vi "UNITEST MAIN v2.0.vi"() -> ()   [LabVIEW 2025] (continued)
      n520 = Bundle By Name(cluster=w613, "New PID LOGIC.Fine Tune Zone"=w611, "New PID LOGIC.PID SDelay"=w610, "New PID LOGIC.Max_pos_limit"=w609, "New PID LOGIC.Min_pos_limit"=w608, "New PID LOGIC.i_limit"=w607, "New PID LOGIC.pct_scale"=w598, "New PID LOGIC.Deadband"=w606, "New PID LOGIC.Kd"=w605, "New PID LOGIC.Ki"=w604, "New PID LOGIC.Kp"=w603, "New PID LOGIC.Current Position"=w602, "New PID LOGIC.Set Load"=w601, "New PID LOGIC.Current Load"=w600, "New PID LOGIC.Pulse delta"=w599, "New PID LOGIC.Init Step"=w597, "New PID LOGIC.Max Step Linit"=w596, "New PID LOGIC.min_deadband_floor"=w595, "New PID LOGIC.dynamic_spindle_noise_scalar"=w594, "New PID LOGIC.min_finetune_floor"=w593, "New PID LOGIC.filter_alpha"=w592, "New PID LOGIC.PID"=w591) -> (w612:T22)
    }
    frame #14 {
      n521 = control-ref of="Manual Write SWAY"() -> (w652:refnum<vi>)
      n522 = control-ref of="Read SWAY Temp"() -> (w633:refnum<vi>)
      n523 = control-ref of="error out Write  SWAY"() -> (w654:refnum<vi>)
      n524 = control-ref of="error out Read SWAY"() -> (w653:refnum<vi>)
      n525 = control-ref of="faultCode Rotary"() -> (w616:refnum<vi>)
      n526 = control-ref of="UPLINK SWAY"() -> (w615:refnum<vi>)
      n527 = control-ref of="DOWNLINK SWAY"() -> (w614:refnum<vi>)
      n528 = control-ref of="fwMajor"() -> (w671:refnum<vi>)
      n529 = control-ref of="Homed"() -> (w670:refnum<vi>)
      n530 = control-ref of="Rotary POSE"() -> (w669:refnum<vi>)
      n531 = control-ref of="State"() -> (w668:refnum<vi>)
      n532 = control-ref of="SWAY POSE"() -> (w667:refnum<vi>)
      n533 = control-ref of="Ack ID"() -> (w666:refnum<vi>)
      n534 = control-ref of="faultCode"() -> (w665:refnum<vi>)
      n535 = control-ref of="Node Id"() -> (w664:refnum<vi>)
      n536 = control-ref of="fwMinor"() -> (w663:refnum<vi>)
      n537 = control-ref of="Spare 6"() -> (w662:refnum<vi>)
      n538 = control-ref of="Spare 5"() -> (w661:refnum<vi>)
      n539 = control-ref of="Spare 4"() -> (w660:refnum<vi>)
      n540 = control-ref of="Spare 3"() -> (w659:refnum<vi>)
      n541 = control-ref of="Spare 2"() -> (w658:refnum<vi>)
      n542 = control-ref of="Spare 1"() -> (w657:refnum<vi>)
      n543 = control-ref of="Spare 7"() -> (w656:refnum<vi>)
      n544 = control-ref of="SPARE  5"() -> (w655:refnum<vi>)
      n545 = control-ref of="SPARE  4"() -> (w650:refnum<vi>)
      n546 = control-ref of="SPARE  3"() -> (w649:refnum<vi>)
      n547 = control-ref of="SPARE 2"() -> (w648:refnum<vi>)
      n548 = control-ref of="SPARE1"() -> (w647:refnum<vi>)
      n549 = control-ref of="Spare 15"() -> (w646:refnum<vi>)
      n550 = control-ref of="Spare 14"() -> (w645:refnum<vi>)
      n551 = control-ref of="Spare 13"() -> (w644:refnum<vi>)
      n552 = control-ref of="Spare 12"() -> (w643:refnum<vi>)
      n553 = control-ref of="Spare 11"() -> (w642:refnum<vi>)
      n554 = control-ref of="Spare 9"() -> (w641:refnum<vi>)
      n555 = control-ref of="Spare 8"() -> (w640:refnum<vi>)
      n556 = control-ref of="SPEED"() -> (w639:refnum<vi>)
      n557 = control-ref of="Distance"() -> (w638:refnum<vi>)
      n558 = control-ref of="Mode Command"() -> (w637:refnum<vi>)
      n559 = control-ref of="Sequence ID"() -> (w636:refnum<vi>)
      n560 = control-ref of="Spare 10"() -> (w634:refnum<vi>)
      n561 = control-ref of="faultCode Sway"() -> (w632:refnum<vi>)
      n562 = control-ref of="Missed Packets"() -> (w631:refnum<vi>)
      n563 = control-ref of="System UPTIME"() -> (w630:refnum<vi>)
      n564 = control-ref of="SPARE 6"() -> (w629:refnum<vi>)
      n565 = control-ref of="SPARE 7"() -> (w628:refnum<vi>)
      n566 = control-ref of="SPARE 9"() -> (w627:refnum<vi>)
      n567 = control-ref of="SPARE 11"() -> (w626:refnum<vi>)
      n568 = control-ref of="SPARE 10"() -> (w625:refnum<vi>)
      n569 = control-ref of="SPARE 8"() -> (w624:refnum<vi>)
      n570 = control-ref of="SPARE 13"() -> (w623:refnum<vi>)
      n571 = control-ref of="SPARE 12"() -> (w622:refnum<vi>)
      n572 = control-ref of="SPARE 17"() -> (w621:refnum<vi>)
      n573 = control-ref of="SPARE 16"() -> (w620:refnum<vi>)
      n574 = control-ref of="SPARE 15"() -> (w619:refnum<vi>)
      n575 = control-ref of="SPARE 14"() -> (w618:refnum<vi>)
      n576 = control-ref of="Reserved"() -> (w617:refnum<vi>)
      n577 = control-ref of="SWAY WRITE"() -> (w651:refnum<vi>)
      n578 = control-ref of="SWAY READ"() -> (w635:refnum<vi>)
      n579 = Bundle By Name(cluster=w673, "SWAY.fwMajor"=w671, "SWAY.Homed"=w670, "SWAY.Rotary POSE"=w669, "SWAY.State"=w668, "SWAY.SWAY POSE"=w667, "SWAY.Ack ID"=w666, "SWAY.faultCode"=w665, "SWAY.Node Id"=w664, "SWAY.fwMinor"=w663, "SWAY.Spare 6"=w662, "SWAY.Spare 5"=w661, "SWAY.Spare 4"=w660, "SWAY.Spare 3"=w659, "SWAY.Spare 2"=w658, "SWAY.Spare 1"=w657, "SWAY.Spare 7"=w656, "SWAY.SPARE  5"=w655, "SWAY.error out Write  SWAY"=w654, "SWAY.error out Read SWAY"=w653, "SWAY.Manual Write SWAY"=w652, "SWAY.SWAY WRITE"=w651, "SWAY.SPARE  4"=w650, "SWAY.SPARE  3"=w649, "SWAY.SPARE 2"=w648, "SWAY.SPARE 1"=w647, "SWAY.Spare 15"=w646, "SWAY.Spare 14"=w645, "SWAY.Spare 13"=w644, "SWAY.Spare 12"=w643, "SWAY.Spare 11"=w642, "SWAY.Spare 9"=w641, "SWAY.Spare 8"=w640, "SWAY.SPEED"=w639, "SWAY.Distance"=w638, "SWAY.Mode Command"=w637, "SWAY.Sequence ID"=w636, "SWAY.SWAY READ"=w635, "SWAY.Spare 10"=w634, "SWAY.Read SWAY Temp"=w633, "SWAY.faultCode Sway"=w632, "SWAY.Missed Packets"=w631, "SWAY.System UPTIME sway"=w630, "SWAY.SPARE 6"=w629, "SWAY.SPARE 7"=w628, "SWAY.SPARE 9"=w627, "SWAY.SPARE 11"=w626, "SWAY.SPARE 10"=w625, "SWAY.SPARE 8"=w624, "SWAY.SPARE 13"=w623, "SWAY.SPARE 12"=w622, "SWAY.SPARE 17"=w621, "SWAY.SPARE 16"=w620, "SWAY.SPARE 15"=w619, "SWAY.SPARE 14"=w618, "SWAY.Reserved"=w617, "SWAY.faultCode Rotary"=w616, "SWAY.UPLINK SWAY"=w615, "SWAY.DOWNLINK SWAY"=w614) -> (w672:T22)
    }
    frame #15 {
      n580 = control-ref of="Analysis Home new"() -> (w704:refnum<vi>)
      n581 = control-ref of="Refresh 2"() -> (w703:refnum<vi>)
      n582 = control-ref of="OPEN 4"() -> (w689:refnum<vi>)
      n583 = control-ref of="OPEN 3"() -> (w687:refnum<vi>)
      n584 = control-ref of="XY Graph"() -> (w682:refnum<vi>)
      n585 = control-ref of="OPEN 2"() -> (w679:refnum<vi>)
      n586 = control-ref of="OPEN 1"() -> (w678:refnum<vi>)
      n587 = control-ref of="Export"() -> (w675:refnum<vi>)
      n588 = control-ref of="MEAN"() -> (w702:refnum<vi>)
      n589 = control-ref of="SD"() -> (w701:refnum<vi>)
      n590 = control-ref of="VARIANCE"() -> (w700:refnum<vi>)
      n591 = control-ref of="MEAN"() -> (w699:refnum<vi>)
      n592 = control-ref of="SD"() -> (w698:refnum<vi>)
      n593 = control-ref of="VARIANCE"() -> (w697:refnum<vi>)
      n594 = control-ref of="MEAN"() -> (w696:refnum<vi>)
      n595 = control-ref of="SD"() -> (w695:refnum<vi>)
      n596 = control-ref of="VARIANCE"() -> (w694:refnum<vi>)
      n597 = control-ref of="MEAN"() -> (w693:refnum<vi>)
      n598 = control-ref of="SD"() -> (w692:refnum<vi>)
      n599 = control-ref of="VARIANCE"() -> (w691:refnum<vi>)
      n600 = control-ref of="File 4 Discription"() -> (w690:refnum<vi>)
      n601 = control-ref of="File Name 4"() -> (w688:refnum<vi>)
      n602 = control-ref of="File 3 Discription"() -> (w686:refnum<vi>)
      n603 = control-ref of="File Name 3"() -> (w685:refnum<vi>)
      n604 = control-ref of="File Name 2"() -> (w681:refnum<vi>)
      n605 = control-ref of="File Name 1"() -> (w680:refnum<vi>)
      n606 = control-ref of="File 1 Discription"() -> (w677:refnum<vi>)
      n607 = control-ref of="File 2 Discription"() -> (w676:refnum<vi>)
      n608 = control-ref of="Y-AXIS"() -> (w684:refnum<vi>)
      n609 = control-ref of="X-AXIS"() -> (w683:refnum<vi>)
      n610 = control-ref of="File Format"() -> (w674:refnum<vi>)
      n611 = Bundle By Name(cluster=w706, "Analysis Screen.Analysis Home"=w704, "Analysis Screen.Refresh 2"=w703, "Analysis Screen.MEAN 4"=w702, "Analysis Screen.SD 4"=w701, "Analysis Screen.VARIANCE 4"=w700, "Analysis Screen.MEAN  3"=w699, "Analysis Screen.SD  3"=w698, "Analysis Screen.VARIANCE  3"=w697, "Analysis Screen.MEAN 2"=w696, "Analysis Screen.SD  2"=w695, "Analysis Screen.VARIANCE 2"=w694, "Analysis Screen.MEAN"=w693, "Analysis Screen.SD"=w692, "Analysis Screen.VARIANCE"=w691, "Analysis Screen.File 4 Discription"=w690, "Analysis Screen.OPEN 4"=w689, "Analysis Screen.File Name 4"=w688, "Analysis Screen.OPEN 3"=w687, "Analysis Screen.File 3 Discription"=w686, "Analysis Screen.File Name 3"=w685, "Analysis Screen.Y-AXIS"=w684, "Analysis Screen.X-AXIS"=w683, "Analysis Screen.XY Graph"=w682, "Analysis Screen.File Name 2"=w681, "Analysis Screen.File Name 1"=w680, "Analysis Screen.OPEN 2"=w679, "Analysis Screen.OPEN 1"=w678, "Analysis Screen.File 1 Discription"=w677, "Analysis Screen.File 2 Discription"=w676, "Analysis Screen.Export"=w675, "Analysis Screen.File Format"=w674) -> (w705:T22)
    }
    frame #16 {
      n612 = control-ref of="Manual Write TRACTION"() -> (w738:refnum<vi>)
      n613 = control-ref of="Read TRACTION Temp"() -> (w725:refnum<vi>)
      n614 = control-ref of="error out Read TRACTION"() -> (w712:refnum<vi>)
      n615 = control-ref of="error out Write  TRACTION"() -> (w711:refnum<vi>)
      n616 = control-ref of="Downlink traction"() -> (w708:refnum<vi>)
      n617 = control-ref of="Uplink Traction"() -> (w707:refnum<vi>)
      n618 = control-ref of="Spare 3"() -> (w709:refnum<vi>)
      n619 = control-ref of="faultCode Traction 2"() -> (w756:refnum<vi>)
      n620 = control-ref of="faultCode Traction 1"() -> (w755:refnum<vi>)
      n621 = control-ref of="Missed Packets"() -> (w754:refnum<vi>)
      n622 = control-ref of="System UPTIME"() -> (w753:refnum<vi>)
      n623 = control-ref of="SPARE 17"() -> (w752:refnum<vi>)
      n624 = control-ref of="SPARE 16"() -> (w751:refnum<vi>)
      n625 = control-ref of="SPARE 15"() -> (w750:refnum<vi>)
      n626 = control-ref of="SPARE 14"() -> (w749:refnum<vi>)
      n627 = control-ref of="SPARE 13"() -> (w748:refnum<vi>)
      n628 = control-ref of="SPARE 12"() -> (w747:refnum<vi>)
      n629 = control-ref of="SPARE 11"() -> (w746:refnum<vi>)
      n630 = control-ref of="SPARE 10"() -> (w745:refnum<vi>)
      n631 = control-ref of="SPARE 9"() -> (w744:refnum<vi>)
      n632 = control-ref of="SPARE 8"() -> (w743:refnum<vi>)
      n633 = control-ref of="SPARE 7"() -> (w742:refnum<vi>)
      n634 = control-ref of="SPARE 6"() -> (w741:refnum<vi>)
      n635 = control-ref of="Reserved"() -> (w740:refnum<vi>)
      n636 = control-ref of="SPARE  5"() -> (w739:refnum<vi>)
      n637 = control-ref of="SPARE  4"() -> (w736:refnum<vi>)
      n638 = control-ref of="SPARE  3"() -> (w735:refnum<vi>)
      n639 = control-ref of="SPARE 2"() -> (w734:refnum<vi>)
      n640 = control-ref of="SPARE 1"() -> (w733:refnum<vi>)
      n641 = control-ref of="Spare 7"() -> (w732:refnum<vi>)
      n642 = control-ref of="Spare 6"() -> (w731:refnum<vi>)
      n643 = control-ref of="Spare 5"() -> (w730:refnum<vi>)
      n644 = control-ref of="Spare 4"() -> (w729:refnum<vi>)
      n645 = control-ref of="Spare 2"() -> (w728:refnum<vi>)
      n646 = control-ref of="Spare 1"() -> (w727:refnum<vi>)
      n647 = control-ref of="Node Id"() -> (w726:refnum<vi>)
      n648 = control-ref of="fwMinor"() -> (w724:refnum<vi>)
      n649 = control-ref of="fwMajor"() -> (w723:refnum<vi>)
      n650 = control-ref of="faultCode"() -> (w722:refnum<vi>)
      n651 = control-ref of="TRACTION POSE 2"() -> (w721:refnum<vi>)
      n652 = control-ref of="TRACTION POSE 1"() -> (w720:refnum<vi>)
      n653 = control-ref of="Homed"() -> (w719:refnum<vi>)
      n654 = control-ref of="State"() -> (w718:refnum<vi>)
      n655 = control-ref of="Ack ID"() -> (w717:refnum<vi>)
      n656 = control-ref of="SPEED"() -> (w716:refnum<vi>)
      n657 = control-ref of="Distance"() -> (w715:refnum<vi>)
      n658 = control-ref of="Mode Command"() -> (w714:refnum<vi>)
      n659 = control-ref of="Sequence ID"() -> (w713:refnum<vi>)
      n660 = control-ref of="TRACTION WRITE"() -> (w737:refnum<vi>)
      n661 = control-ref of="TRACTION READ"() -> (w710:refnum<vi>)
      n662 = Bundle By Name(cluster=w758, "Traction.faultCode Traction 2"=w756, "Traction.faultCode Traction 1"=w755, "Traction.Missed Packets"=w754, "Traction.System UPTIME Traction"=w753, "Traction.SPARE 17"=w752, "Traction.SPARE 16"=w751, "Traction.SPARE 15"=w750, "Traction.SPARE 14"=w749, "Traction.SPARE 13"=w748, "Traction.SPARE 12"=w747, "Traction.SPARE 11"=w746, "Traction.SPARE 10"=w745, "Traction.SPARE 9"=w744, "Traction.SPARE 8"=w743, "Traction.SPARE 7"=w742, "Traction.SPARE 6"=w741, "Traction.Reserved"=w740, "Traction.SPARE  5"=w739, "Traction.Manual Write TRACTION"=w738, "Traction.TRACTION WRITE"=w737, "Traction.SPARE  4"=w736, "Traction.SPARE  3"=w735, "Traction.SPARE 2"=w734, "Traction.SPARE 1"=w733, "Traction.Spare 7"=w732, "Traction.Spare 6"=w731, "Traction.Spare 5"=w730, "Traction.Spare 4"=w729, "Traction.Spare 2"=w728, "Traction.Spare 1"=w727, "Traction.Node Id"=w726, "Traction.Read TRACTION Temp"=w725, "Traction.fwMinor"=w724, "Traction.fwMajor"=w723, "Traction.faultCode"=w722, "Traction.TRACTION POSE"=w721, "Traction.TRACTION POSE 2"=w720, "Traction.Homed"=w719, "Traction.State"=w718, "Traction.Ack ID"=w717, "Traction.SPEED"=w716, "Traction.Distance"=w715, "Traction.Mode Command"=w714, "Traction.Sequence ID"=w713, "Traction.error out Read TRACTION"=w712, "Traction.error out Write  TRACTION"=w711, "Traction.TRACTION READ"=w710, "Traction.Spare 3"=w709, "Traction.Downlink traction"=w708, "Traction.Uplink Traction"=w707) -> (w757:T22)
    }
    frame #17 {
      n663 = control-ref of="Traction Receipe"() -> (w780:refnum<vi>)
      n664 = control-ref of="Total Execution Time"() -> (w791:refnum<vi>)
      n665 = control-ref of="Total Steps"() -> (w790:refnum<vi>)
      n666 = control-ref of="Duration / Step (s)"() -> (w789:refnum<vi>)
      n667 = control-ref of="Duration / Step (s)"() -> (w787:refnum<vi>)
      n668 = control-ref of="Speed (mm/s)"() -> (w785:refnum<vi>)
      n669 = control-ref of="SET entrainment Velocity"() -> (w779:refnum<vi>)
      n670 = control-ref of="Test Array Size"() -> (w778:refnum<vi>)
      n671 = control-ref of="SRR INDEX [ STRIBECK]"() -> (w777:refnum<vi>)
      n672 = control-ref of="Stribeck Size"() -> (w776:refnum<vi>)
      n673 = control-ref of="SET SRR"() -> (w775:refnum<vi>)
      n674 = control-ref of="ELAPSED TIMER"() -> (w774:refnum<vi>)
      n675 = control-ref of="BALL SET RPM"() -> (w773:refnum<vi>)
      n676 = control-ref of="DISC SET RPM"() -> (w772:refnum<vi>)
      n677 = control-ref of="SET LOAD"() -> (w771:refnum<vi>)
      n678 = control-ref of="TEMPERATURE READ"() -> (w770:refnum<vi>)
      n679 = control-ref of="SET TEMPERATURE"() -> (w769:refnum<vi>)
      n680 = control-ref of="Traction Size"() -> (w768:refnum<vi>)
      n681 = control-ref of="DISC SPEED (rpm)"() -> (w767:refnum<vi>)
      n682 = control-ref of="BALL SPEED (rpm)"() -> (w766:refnum<vi>)
      n683 = control-ref of="BALL WEAR TRACK"() -> (w765:refnum<vi>)
      n684 = control-ref of="DISC WEARTRACK"() -> (w764:refnum<vi>)
      n685 = control-ref of="SRR INDEX [ TRACTION]"() -> (w763:refnum<vi>)
      n686 = control-ref of="Start Index Type"() -> (w762:refnum<vi>)
      n687 = control-ref of="Ball (mm/sec)"() -> (w760:refnum<vi>)
      n688 = control-ref of="Disc (mm/sec)"() -> (w759:refnum<vi>)
      n689 = control-ref of="SRR Sweep Range (%)"() -> (w792:refnum<vi>)
      n690 = control-ref of="STRIBECK Fixed SRR List (%)"() -> (w788:refnum<vi>)
      n691 = control-ref of="SRR Sweep Range (%)"() -> (w786:refnum<vi>)
      n692 = control-ref of="Temperature Stages (°C)"() -> (w784:refnum<vi>)
      n693 = control-ref of="Load (N)"() -> (w783:refnum<vi>)
      n694 = control-ref of="Lubricant Name"() -> (w782:refnum<vi>)
      n695 = control-ref of="Profile File Name"() -> (w781:refnum<vi>)
      n696 = control-ref of="Enum - Menu"() -> (w761:refnum<vi>)
      n697 = Bundle By Name(cluster=w794, "Traction reciepe.SRR Sweep Range (%) Stribeck"=w792, "Traction reciepe.Traction Receipe"=w780, "Traction reciepe.Total Execution Time"=w791, "Traction reciepe.Total Steps"=w790, "Traction reciepe.Duration / Step (s)  Stribeck"=w789, "Traction reciepe.STRIBECK Fixed SRR List (%)"=w788, "Traction reciepe.Duration / Step (s) Traction"=w787, "Traction reciepe.SRR Sweep Range (%) traction"=w786, "Traction reciepe.Rolling Speed (mm/s)"=w785, "Traction reciepe.Temperature Stages (°C)"=w784, "Traction reciepe.Ball Load (N)"=w783, "Traction reciepe.Lubricant Name"=w782, "Traction reciepe.Profile File Name"=w781, "Traction reciepe.SET entrainment Velocity"=w779, "Traction reciepe.Test Array Size"=w778, "Traction reciepe.SRR INDEX [ STRIBECK]"=w777, "Traction reciepe.Stribeck Size"=w776, "Traction reciepe.SET SRR"=w775, "Traction reciepe.ELAPSED TIMER"=w774, "Traction reciepe.BALL SET RPM"=w773, "Traction reciepe.DISC SET RPM"=w772, "Traction reciepe.SET LOAD"=w771, "Traction reciepe.TEMPERATURE READ"=w770, "Traction reciepe.SET TEMPERATURE"=w769, "Traction reciepe.Traction Size"=w768, "Traction reciepe.DISC SPEED (rpm)"=w767, "Traction reciepe.BALL SPEED (rpm)"=w766, "Traction reciepe.BALL WEAR TRACK"=w765, "Traction reciepe.DISC WEARTRACK"=w764, "Traction reciepe.SRR INDEX [ TRACTION]"=w763, "Traction reciepe.Start Index Type"=w762, "Traction reciepe.Enum - Menu"=w761, "Traction reciepe.Ball (mm/sec)"=w760, "Traction reciepe.Disc (mm/sec)"=w759) -> (w793:T22)
    }
    frame #18 {
      n698 = control-ref of="SPEED SELECTION : MTM"() -> (w823:refnum<vi>)
      n699 = control-ref of="TEST SELECTION (MTM)"() -> (w822:refnum<vi>)
      n700 = control-ref of="MTM Test Selection"() -> (w821:refnum<vi>)
      n701 = control-ref of="TEST SELECTION (MTM) 2"() -> (w809:refnum<vi>)
      n702 = control-ref of="SPEED SELECTION : MTM 2"() -> (w808:refnum<vi>)
      n703 = control-ref of="MTM Test Selection 2"() -> (w807:refnum<vi>)
      n704 = control-ref of="Demo Mode Display"() -> (w851:refnum<vi>)
      n705 = control-ref of="Main Tab sequence for selection"() -> (w848:refnum<vi>)
      n706 = control-ref of="Ramp Tab"() -> (w847:refnum<vi>)
      n707 = control-ref of="e.v/ssr"() -> (w846:refnum<vi>)
      n708 = control-ref of="File Path Tab"() -> (w820:refnum<vi>)
      n709 = control-ref of="Step Sequence Indication Tab"() -> (w815:refnum<vi>)
      n710 = control-ref of="Disc Speed Indicator"() -> (w796:refnum<vi>)
      n711 = control-ref of="HomeTraction"() -> (w852:refnum<vi>)
      n712 = control-ref of="Traction Step Update Details"() -> (w849:refnum<vi>)
      n713 = control-ref of="E.Velocity"() -> (w838:refnum<vi>)
      n714 = control-ref of="Ramp Up   Disc"() -> (w835:refnum<vi>)
      n715 = control-ref of="Ramp Up"() -> (w828:refnum<vi>)
      n716 = control-ref of="BallSpeed Exceed Indication"() -> (w825:refnum<vi>)
      n717 = control-ref of="Apply"() -> (w824:refnum<vi>)
      n718 = control-ref of="Save"() -> (w818:refnum<vi>)
      n719 = control-ref of="Import"() -> (w817:refnum<vi>)
      n720 = control-ref of="Calculate Step"() -> (w813:refnum<vi>)
      n721 = control-ref of="Enter Fixed E.Velocity"() -> (w845:refnum<vi>)
      n722 = control-ref of="Enter Final SRR"() -> (w844:refnum<vi>)
      n723 = control-ref of="Enter initial SRR"() -> (w843:refnum<vi>)
      n724 = control-ref of="Enter Fixed SRR"() -> (w842:refnum<vi>)
      n725 = control-ref of="Enter the Final E.Velocity (m/s)"() -> (w841:refnum<vi>)
      n726 = control-ref of="Enter initial E.Velocity (m/s)"() -> (w840:refnum<vi>)
      n727 = control-ref of="Ball WTD"() -> (w839:refnum<vi>)
      n728 = control-ref of="Enter the Final Velocity (m/s)"() -> (w837:refnum<vi>)
      n729 = control-ref of="Enter initial Velocity (m/s)"() -> (w836:refnum<vi>)
      n730 = control-ref of="Initial DiscSpeed (RPM)"() -> (w834:refnum<vi>)
      n731 = control-ref of="Final Speed (RPM)"() -> (w833:refnum<vi>)
      n732 = control-ref of="Final Speed (RPM) Ball"() -> (w832:refnum<vi>)
      n733 = control-ref of="Initial Speed (RPM) Ball"() -> (w831:refnum<vi>)
      n734 = control-ref of="Enter the Final Velocity (m/s) Ball"() -> (w830:refnum<vi>)
      n735 = control-ref of="Enter initial Velocity (m/s) Ball"() -> (w829:refnum<vi>)
      n736 = control-ref of="Enter the Speed (m/sec):"() -> (w806:refnum<vi>)
      n737 = control-ref of="Enter the Speed (m/sec):"() -> (w805:refnum<vi>)
      n738 = control-ref of="Enter the Speed (RPM):"() -> (w804:refnum<vi>)
      n739 = control-ref of="Enter the Speed (RPM):Ball"() -> (w801:refnum<vi>)
      n740 = control-ref of="Wear Track Diameter (mm)"() -> (w797:refnum<vi>)
      n741 = control-ref of="ExceedBallSpeed"() -> (w795:refnum<vi>)
      n742 = control-ref of="Traction Message"() -> (w850:refnum<vi>)
      n743 = control-ref of="ExceedBallSpeed step"() -> (w827:refnum<vi>)
      n744 = control-ref of="ExceedDiscSpeed"() -> (w826:refnum<vi>)
      n745 = control-ref of="File Path String"() -> (w819:refnum<vi>)
      n746 = control-ref of="Step Sequence Indication"() -> (w814:refnum<vi>)
      n747 = control-ref of="ExceedDiscSpeed  Cinstant Speed"() -> (w811:refnum<vi>)
      n748 = control-ref of="ExceedBallSpeed Constant"() -> (w810:refnum<vi>)
      n749 = control-ref of="Lower Spped"() -> (w803:refnum<vi>)
      n750 = control-ref of="Upper"() -> (w802:refnum<vi>)
      n751 = control-ref of="StepTable"() -> (w812:refnum<vi>)
      n752 = control-ref of="Disc Motion Direction:"() -> (w800:refnum<vi>)
      n753 = control-ref of="Ball Motion Direction :"() -> (w799:refnum<vi>)
      n754 = control-ref of="Motion Mode:"() -> (w798:refnum<vi>)
      n755 = control-ref of="File Path :"() -> (w816:refnum<vi>)
      n756 = Bundle By Name(cluster=w854, "Traction Control.HomeTraction"=w852, "Traction Control.Demo Mode Display"=w851, "Traction Control.Traction Message"=w850, "Traction Control.Traction Step Update Details"=w849, "Traction Control.Main Tab sequence for selection"=w848, "Traction Control.Ramp Tab"=w847, "Traction Control.e.v/ssr"=w846, "Traction Control.Enter Fixed E.Velocity"=w845, "Traction Control.Enter Final SRR"=w844, "Traction Control.Enter initial SRR"=w843, "Traction Control.Enter Fixed SRR"=w842, "Traction Control.Enter the Final E.Velocity (m/s)"=w841, "Traction Control.Enter initial E.Velocity (m/s)"=w840, "Traction Control.Ball WTD"=w839, "Traction Control.E.Velocity"=w838, "Traction Control.Enter the Final Velocity (m/s)"=w837, "Traction Control.Enter initial Velocity (m/s)"=w836, "Traction Control.Ramp Up   Disc"=w835, "Traction Control.Initial DiscSpeed (RPM)"=w834, "Traction Control.Final Speed (RPM) Ball"=w833, "Traction Control.Final Speed (RPM)"=w832, "Traction Control.Initial Speed (RPM) Ball"=w831, "Traction Control.Enter the Final Velocity (m/s) Ball"=w830, "Traction Control.Enter initial Velocity (m/s) Ball"=w829, "Traction Control.Ramp Up"=w828, "Traction Control.ExceedBallSpeed step"=w827, "Traction Control.ExceedDiscSpeed"=w826, "Traction Control.BallSpeed Exceed Indication"=w825, "Traction Control.Apply"=w824, "Traction Control.SPEED SELECTION : MTM"=w823, "Traction Control.TEST SELECTION (MTM)"=w822, "Traction Control.MTM Test Selection"=w821, "Traction Control.File Path Tab"=w820, "Traction Control.File Path String"=w819, "Traction Control.Save"=w818, "Traction Control.Import"=w817, "Traction Control.File Path :"=w816, "Traction Control.Step Sequence Indication Tab"=w815, "Traction Control.Step Sequence Indication"=w814, "Traction Control.Calculate Step"=w813, "Traction Control.StepTable"=w812, "Traction Control.ExceedDiscSpeed  Cinstant Speed"=w811, "Traction Control.ExceedBallSpeed Constant"=w810, "Traction Control.TEST SELECTION (MTM) 2"=w809, "Traction Control.SPEED SELECTION : MTM 3"=w808, "Traction Control.MTM Test Selection 2"=w807, "Traction Control.Enter the Speed (m/sec):"=w806, "Traction Control.Enter the Speed (m/sec):  2"=w805, "Traction Control.Enter the Speed (RPM):"=w804, "Traction Control.Lower Spped"=w803, "Traction Control.Upper"=w802, "Traction Control.Enter the Speed (RPM):Ball"=w801, "Traction Control.Disc Motion Direction:"=w800, "Traction Control.Ball Motion Direction :"=w799, "Traction Control.Motion Mode:"=w798, "Traction Control.Wear Track Diameter (mm)"=w797, "Traction Control.Disc Speed Indicator"=w796, "Traction Control.ExceedBallSpeed"=w795) -> (w853:T22)
    }
    frame #19 {
      n757 = control-ref of="Gains"() -> (w856:refnum<vi>)
      n758 = control-ref of="Signal Energy"() -> (w860:refnum<vi>)
      n759 = control-ref of="Amplitude db_AE"() -> (w859:refnum<vi>)
      n760 = control-ref of="Peak Amplitude"() -> (w858:refnum<vi>)
      n761 = control-ref of="AE Ring-Down Counts"() -> (w857:refnum<vi>)
      n762 = control-ref of="Manual Write Acquostic"() -> (w855:refnum<vi>)
      n763 = control-ref of="error out"() -> (w865:refnum<vi>)
      n764 = control-ref of="error in (no error)"() -> (w864:refnum<vi>)
      n765 = control-ref of="Downlink Packet"() -> (w863:refnum<vi>)
      n766 = control-ref of="Uplink Packet"() -> (w862:refnum<vi>)
      n767 = control-ref of="Last Config Rejected"() -> (w870:refnum<vi>)
      n768 = control-ref of="rx command count"() -> (w869:refnum<vi>)
      n769 = control-ref of="Current Filter Id"() -> (w868:refnum<vi>)
      n770 = control-ref of="Isolated Gain"() -> (w867:refnum<vi>)
      n771 = control-ref of="DAQ Status"() -> (w866:refnum<vi>)
      n772 = control-ref of="data out"() -> (w861:refnum<vi>)
      n773 = Bundle By Name(cluster=w872, "Acquostic.Last Config Rejected"=w870, "Acquostic.rx command count"=w869, "Acquostic.Current Filter Id"=w868, "Acquostic.Isolated Gain"=w867, "Acquostic.DAQ Status"=w866, "Acquostic.error out"=w865, "Acquostic.error in (no error)"=w864, "Acquostic.Downlink Packet"=w863, "Acquostic.Uplink Packet"=w862, "Acquostic.data out"=w861, "Acquostic.Signal Energy"=w860, "Acquostic.Amplitude db_AE"=w859, "Acquostic.Peak Amplitude"=w858, "Acquostic.AE Ring-Down Counts"=w857, "Acquostic.Gains"=w856, "Acquostic.Manual Write Acquostic"=w855) -> (w871:T22)
    }
  }
  n774 = call <userlib>:"Fit VI window to Largest Dec.vi"() -> ("error out"=w57:errorcluster, "dup VI Ref"=w54:refnum<vi>)  [unwired: 6 in]
  n775 = invoke on="Invoke Node" class="VI" method="FP.Run-Time Position.Maximized"(reference=w54, error in=w57) -> (error out=w56:errorcluster)  [unwired: 2 in, 3 out]
  n776 = call <vilib>:"Clear Errors.vi"("error in (no error)"=w56) -> ("error out"=w55:errorcluster)  [unwired: 5 in, 1 out]
  n777 = control-ref of="This VI"() -> (w60:refnum<vi>)
  n778 = invoke on="Invoke Node" class="VI" method="Default Vals.Reinit All"(reference=w60, error in=w55) -> (reference out=w58:refnum<vi>, error out=w59:errorcluster)  [unwired: 1 in, 1 out]
  n779 = Close Reference(reference=w58, error in (no error)=w59) -> (error out=w53:errorcluster)
  n780 = call "Create User Event - Stop.vi"("error in (no error)"=w53) -> ("error out"=w6:errorcluster, "User Event - Stop"=w10:refnum<user-event>)  [unwired: 9 in]
  n781 = call "main screen queue out Unitest.vi"("error in (no error)"=w6) -> ("error out"=w80:errorcluster, "output Queue"=w8:T23)  [unwired: 9 in]
  n782 = Unbundle By Name(w8) -> ("RAMP MOTOR COM LOOP"=w46:refnum<queue>)
  n783 = Unbundle By Name(w8) -> ("TEMPERATURE COM LOOP"=w48:refnum<queue>)
  n784 = Unbundle By Name(w8) -> ("ECR PORT"=w45:refnum<queue>)
  n785 = Unbundle By Name(w8) -> ("SWAY MOTOR COM LOOP"=w50:refnum<queue>)
  n786 = Unbundle By Name(w8) -> ("UI Loop"=w78:refnum<queue>)
  n787 = Unbundle By Name(w8) -> ("LOAD COM LOOP"=w51:refnum<queue>)
  n788 = Unbundle By Name(w8) -> ("HEAVE MOTOR COM LOOP"=w35:refnum<queue>)
  n789 = Unbundle By Name(w8) -> ("HUMIDITY COM PORT"=w44:refnum<queue>)
  n790 = Unbundle By Name(w8) -> ("PROGRAM LOOP"=w43:refnum<queue>)
  n791 = Unbundle By Name(w8) -> ("MONITOR LOOP"=w42:refnum<queue>)
  n792 = Unbundle By Name(w8) -> ("LOAD PID"=w41:refnum<queue>)
  n793 = Unbundle By Name(w8) -> ("REPORT"=w40:refnum<queue>)
  n794 = register-events(w10) -> (reference out=w72:refnum<event-registration>, error out=w70:errorcluster)  [unwired: 2 in]
  n795 = Unbundle By Name(w8) -> ("ACOUSTIC"=w7:refnum<queue>)
  n796 = Merge Errors(w70, w80) -> (w71:errorcluster)
  n797 = node-c288() -> (w26:T24)  [unwired: 4 in]
  n798 = node-c288() -> (w4:T24)  [unwired: 4 in]
  n799 = node-c288() -> (w20:T24)  [unwired: 6 in]
  n800 = node-c288() -> (w28:T24)  [unwired: 4 in]
  n801 = node-c288() -> (w30:T24)  [unwired: 4 in]
  n802 = node-c288() -> (w2:T24)  [unwired: 4 in]
  n803 = disable-structure "Diagram Disable Structure" shown="Disabled" {
    disable-tunnel: w44 -> [w877 _]
    disable-tunnel: w9 -> [w876 _]
    disable-tunnel: w10 -> [w875 _]
    disable-tunnel: w6 -> [w874 _]
    disable-tunnel: [w873 _] -> w16
    frame Disabled {
      n804 = while {
        shift-right: [w888] -> _
        shift-left: w876 -> [w889]
        tunnel: [w882] -> w873
        tunnel: w877 -> [w880]
        tunnel: w874 -> [w879]
        tunnel: w875 -> [w878]
        stop <- w887 stop-if-true
        # "Humidity  Handling Loop"
        n805 = call "Dequeue Message.vi"("error in (no error)"=w879, "Message Queue"=w880) -> ("error out"=w886:errorcluster, "Message Data"=w884:variant, "Message"=w885:string, "dup Message Queue"=w883:refnum<queue>)  [unwired: 6 in]
        n806 = case "Message Cases" shown="\"Humidity Main\"" w885 {
          selector: w885 -> [_ _ _ _ _ w933]
          tunnel: w883 -> [w890 w901 _ w920 w932 _]
          tunnel: w886 -> [w893 w898 w917 w924 w926 _]
          tunnel: [w894 w902 w911 w922 w928 w934] -> w881
          tunnel: w889 -> [w892 w900 w916 w923 w931 w935]
          tunnel: [w892 w900 w916 w923 w931 w935] -> w888
          tunnel: [_ _ _ _ TRUE _] -> w887
          tunnel: w884 -> [_ _ w915 _ _ _]
          tunnel: w878 -> [_ _ _ _ w925 _]
          frame "init" {
            # "Initialize - All initialization work should take place in this message, since other loops can potentially enqueue messages that execute immediately after this one."
            n807 = call-poly "Enqueue Message.vi"("error in (no error)"=w893, "Message"="Humidity Main", "Message Queue"=w890) -> ("error out"=w894:errorcluster)  [unwired: 7 in, 1 out]
          }
          frame "Humidity Main" {
            n808 = Unbundle By Name(w900) -> ("Main Home Screen.EXIT"=w899:refnum<vi>)
            n809 = property on="Property Node" class="Bool (strict)"(reference=w899) -> (reference out=w896:refnum<vi>, error out=w897:errorcluster, "Value"=w895:bool)  [unwired: 1 in]
            n810 = case shown="False" w895 {
              tunnel: [w905 w909] -> w902
              tunnel: w901 -> [w904 w908]
              tunnel: w898 -> [w903 w907]
              frame True {
                n811 = call-poly "Enqueue Message.vi"("error in (no error)"=w903, "Message"="Confirm Quit", "Message Queue"=w904) -> ("error out"=w905:errorcluster)  [unwired: 7 in, 1 out]
              }
              frame False {
                n812 = call-poly "Enqueue Message.vi"("error in (no error)"=w907, "Message"="Humidity Main", "Message Queue"=w908) -> ("error out"=w909:errorcluster)  [unwired: 7 in, 1 out]
              }
            }
            n813 = Close Reference(reference=w896, error in (no error)=w897) -> ()  [unwired: 1 out]
          }
          frame "Error" {
            # "#CodeRecommended - If you ever change the name of this \"Error\" message, you'll need to update the name in the Check Loop Error.vi as well."
            # "#CodeRecommended - Consider creating a system for logging errors in some way. These errors are for notification purposes only. Handling of specific errors should be performed in the message frames that generated the error."
            # "Error - Display an error dialog. This message is sent by the \"Error Handler\" VIs at the end of other loops in this application."
            n814 = Variant To Data(error in=w917, type=errorcluster {"status"=FALSE, "code"=0, "source"=""} ("error constant"), Variant=w915) -> (data=w913:errorcluster, error out=w912:errorcluster)
            n815 = call <vilib>:"Simple Error Handler.vi"("error in (no error)"=w913) -> ()  [unwired: 4 in, 5 out]
            n816 = Merge Errors(w912) -> (w911:errorcluster)
          }
          frame "Confirm Quit" {
            # "#CodeNeeded - If you want to provide an \"Are you sure\" dialog (or some other notification) before the application exits, place that code here. This message is typically sent from a Panel Close? event."
            # "Confirm Quit - Message that can confirm whether or not the user wants to exit the application."
            n817 = call-poly "Enqueue Message.vi"("Priority Message? (F)"=TRUE, "error in (no error)"=w924, "Message"="Exit", "Message Queue"=w920) -> ("error out"=w921:errorcluster)  [unwired: 6 in, 1 out]
            n818 = Merge Errors(w921) -> (w922:errorcluster)
          }
          frame "Exit" {
            # "Stop the VI"
            # "Release the message queue reference"
            # "#CodeNeeded - Add any required cleanup code here. Note that if 'Exit' was called as a result of an error, an error dialog will be displayed. Add any custom error handling for an 'Exit' condition here as well."
            # "Exit - Exit the application."
            n819 = call "Fire User Event - Stop.vi"("User Event - Stop"=w925) -> ("error out"=w927:errorcluster)  [unwired: 10 in]
            n820 = Release Queue(queue=w932, error in (no error)=w926) -> (error out=w929:errorcluster)  [unwired: 1 in, 2 out]
            n821 = Merge Errors(w927, w929) -> (w928:errorcluster)
          }
          frame Default {
            # "'Default' case only runs if there is a message that isn't defined in any of the other cases.  Output a programming error."
            n822 = xnode ("Error Ring")("parameter 0"=w933) -> ("error out"=w934:errorcluster)
          }
        }
        n823 = call "LAB-IQ Error Handler - Message Handling Loop.vi"("error in (no error)"=w881, "Message Queue"=w883) -> ("dup error in"=w882:errorcluster)  [unwired: 8 in, 1 out]
      }
    }
    frame Enabled {
    }
  }
  n824 = disable-structure "Diagram Disable Structure" shown="Disabled" {
    disable-tunnel: w45 -> [w947 _]
    disable-tunnel: w9 -> [w946 _]
    disable-tunnel: w10 -> [w945 _]
    disable-tunnel: w6 -> [w944 w1013]
    disable-tunnel: [w943 w1013] -> w17
    frame Disabled {
      n825 = while {
        shift-right: [w958] -> _
        shift-left: w946 -> [w959]
        tunnel: [w952] -> w943
        tunnel: w947 -> [w950]
        tunnel: w944 -> [w949]
        tunnel: w945 -> [w948]
        stop <- w957 stop-if-true
        # "ECR  Handling Loop"
        n826 = call "Dequeue Message.vi"("error in (no error)"=w949, "Message Queue"=w950) -> ("error out"=w956:errorcluster, "Message Data"=w954:variant, "Message"=w955:string, "dup Message Queue"=w953:refnum<queue>)  [unwired: 6 in]
        n827 = case "Message Cases" shown="\"ECR Main\"" w955 {
          selector: w955 -> [_ _ _ _ _ w1003]
          tunnel: w953 -> [w960 w971 _ w990 w1002 _]
          tunnel: w956 -> [w963 w968 w987 w994 w996 _]
          tunnel: [w964 w972 w981 w992 w998 w1004] -> w951
          tunnel: w959 -> [w962 w970 w986 w993 w1001 w1005]
          tunnel: [w962 w970 w986 w993 w1001 w1005] -> w958
          tunnel: [_ _ _ _ TRUE _] -> w957
          tunnel: w954 -> [_ _ w985 _ _ _]
          tunnel: w948 -> [_ _ _ _ w995 _]
          frame "init" {
            # "Initialize - All initialization work should take place in this message, since other loops can potentially enqueue messages that execute immediately after this one."
            n828 = call-poly "Enqueue Message.vi"("error in (no error)"=w963, "Message"="ECR Main", "Message Queue"=w960) -> ("error out"=w964:errorcluster)  [unwired: 7 in, 1 out]
          }
          frame "ECR Main" {
            n829 = Unbundle By Name(w970) -> ("Main Home Screen.EXIT"=w969:refnum<vi>)
            n830 = property on="Property Node" class="Bool (strict)"(reference=w969) -> (reference out=w966:refnum<vi>, error out=w967:errorcluster, "Value"=w965:bool)  [unwired: 1 in]
            n831 = case shown="False" w965 {
              tunnel: [w975 w979] -> w972
              tunnel: w971 -> [w974 w978]
              tunnel: w968 -> [w973 w977]
              frame True {
                n832 = call-poly "Enqueue Message.vi"("error in (no error)"=w973, "Message"="Confirm Quit", "Message Queue"=w974) -> ("error out"=w975:errorcluster)  [unwired: 7 in, 1 out]
              }
              frame False {
                n833 = call-poly "Enqueue Message.vi"("error in (no error)"=w977, "Message"="ECR Main", "Message Queue"=w978) -> ("error out"=w979:errorcluster)  [unwired: 7 in, 1 out]
              }
            }
            n834 = Close Reference(reference=w966, error in (no error)=w967) -> ()  [unwired: 1 out]
          }
          frame "Error" {
            # "#CodeRecommended - If you ever change the name of this \"Error\" message, you'll need to update the name in the Check Loop Error.vi as well."
            # "#CodeRecommended - Consider creating a system for logging errors in some way. These errors are for notification purposes only. Handling of specific errors should be performed in the message frames that generated the error."
            # "Error - Display an error dialog. This message is sent by the \"Error Handler\" VIs at the end of other loops in this application."
            n835 = Variant To Data(error in=w987, type=errorcluster {"status"=FALSE, "code"=0, "source"=""} ("error constant"), Variant=w985) -> (data=w983:errorcluster, error out=w982:errorcluster)
            n836 = call <vilib>:"Simple Error Handler.vi"("error in (no error)"=w983) -> ()  [unwired: 4 in, 5 out]
            n837 = Merge Errors(w982) -> (w981:errorcluster)
          }
          frame "Confirm Quit" {
            # "#CodeNeeded - If you want to provide an \"Are you sure\" dialog (or some other notification) before the application exits, place that code here. This message is typically sent from a Panel Close? event."
            # "Confirm Quit - Message that can confirm whether or not the user wants to exit the application."
            n838 = call-poly "Enqueue Message.vi"("Priority Message? (F)"=TRUE, "error in (no error)"=w994, "Message"="Exit", "Message Queue"=w990) -> ("error out"=w991:errorcluster)  [unwired: 6 in, 1 out]
            n839 = Merge Errors(w991) -> (w992:errorcluster)
          }
          frame "Exit" {
            # "Stop the VI"
            # "Release the message queue reference"
            # "#CodeNeeded - Add any required cleanup code here. Note that if 'Exit' was called as a result of an error, an error dialog will be displayed. Add any custom error handling for an 'Exit' condition here as well."
            # "Exit - Exit the application."
            n840 = call "Fire User Event - Stop.vi"("User Event - Stop"=w995) -> ("error out"=w997:errorcluster)  [unwired: 10 in]
            n841 = Release Queue(queue=w1002, error in (no error)=w996) -> (error out=w999:errorcluster)  [unwired: 1 in, 2 out]
            n842 = Merge Errors(w997, w999) -> (w998:errorcluster)
          }
          frame Default {
            # "'Default' case only runs if there is a message that isn't defined in any of the other cases.  Output a programming error."
            n843 = xnode ("Error Ring")("parameter 0"=w1003) -> ("error out"=w1004:errorcluster)
          }
        }
        n844 = call "LAB-IQ Error Handler - Message Handling Loop.vi"("error in (no error)"=w951, "Message Queue"=w953) -> ("dup error in"=w952:errorcluster)  [unwired: 8 in, 1 out]
      }
    }
    frame Enabled {
    }
  }
  n845 = while "Timed Loop" {
    shift-right: [w1015] -> _
    shift-left: w9 -> [w1034]
    tunnel: [w1028] -> w13
    tunnel: w40 -> [w1026]
    tunnel: w6 -> [w1025]
    tunnel: w10 -> [w1024]
    stop <- w1033 stop-if-true
    # "Report  Handling Loop"
    n846 = call "Dequeue Message.vi"("error in (no error)"=w1025, "Message Queue"=w1026) -> ("error out"=w1032:errorcluster, "Message Data"=w1030:variant, "Message"=w1031:string, "dup Message Queue"=w1029:refnum<queue>)  [unwired: 6 in]
    n847 = case "Message Cases" shown="\"Report Main\"" w1031 {
      selector: w1031 -> [_ _ _ _ _ w1079]
      tunnel: w1029 -> [w1035 w1047 _ w1066 w1078 _]
      tunnel: w1032 -> [w1038 w1045 w1063 w1070 w1072 _]
      tunnel: [w1039 w1048 w1057 w1068 w1074 w1080] -> w1027
      tunnel: w1034 -> [w1037 w1040 w1062 w1069 w1077 w1081]
      tunnel: [w1037 w1040 w1062 w1069 w1077 w1081] -> w1015
      tunnel: [_ _ _ _ TRUE _] -> w1033
      tunnel: w1030 -> [_ _ w1061 _ _ _]
      tunnel: w1024 -> [_ _ _ _ w1071 _]
      frame "init" {
        # "Initialize - All initialization work should take place in this message, since other loops can potentially enqueue messages that execute immediately after this one."
        n848 = call-poly "Enqueue Message.vi"("error in (no error)"=w1038, "Message"="Report Main", "Message Queue"=w1035) -> ("error out"=w1039:errorcluster)  [unwired: 7 in, 1 out]
      }
      frame "Report Main" {
        n849 = call "Main Data Log.vi"("error in (no error)"=w1045, "main ref"=w1040) -> ("error out"=w1041:errorcluster)  [unwired: 9 in]
        n850 = Unbundle By Name(w1040) -> ("Main Home Screen.EXIT"=w1046:refnum<vi>)
        n851 = property on="Property Node" class="Bool (strict)"(reference=w1046) -> (reference out=w1043:refnum<vi>, error out=w1044:errorcluster, "Value"=w1042:bool)  [unwired: 1 in]
        n852 = case shown="False" w1042 {
          tunnel: [w1051 w1055] -> w1048
          tunnel: w1047 -> [w1050 w1054]
          tunnel: w1041 -> [w1049 w1053]
          frame True {
            n853 = call-poly "Enqueue Message.vi"("error in (no error)"=w1049, "Message"="Confirm Quit", "Message Queue"=w1050) -> ("error out"=w1051:errorcluster)  [unwired: 7 in, 1 out]
          }
          frame False {
            n854 = call-poly "Enqueue Message.vi"("error in (no error)"=w1053, "Message"="Report Main", "Message Queue"=w1054) -> ("error out"=w1055:errorcluster)  [unwired: 7 in, 1 out]
          }
        }
        n855 = Close Reference(reference=w1043, error in (no error)=w1044) -> ()  [unwired: 1 out]
      }
      frame "Error" {
        # "#CodeRecommended - If you ever change the name of this \"Error\" message, you'll need to update the name in the Check Loop Error.vi as well."
        # "#CodeRecommended - Consider creating a system for logging errors in some way. These errors are for notification purposes only. Handling of specific errors should be performed in the message frames that generated the error."
        # "Error - Display an error dialog. This message is sent by the \"Error Handler\" VIs at the end of other loops in this application."
        n856 = Variant To Data(error in=w1063, type=errorcluster {"status"=FALSE, "code"=0, "source"=""} ("error constant"), Variant=w1061) -> (data=w1059:errorcluster, error out=w1058:errorcluster)
        n857 = call <vilib>:"Simple Error Handler.vi"("error in (no error)"=w1059) -> ()  [unwired: 4 in, 5 out]
        n858 = Merge Errors(w1058) -> (w1057:errorcluster)
      }
      frame "Confirm Quit" {
        # "#CodeNeeded - If you want to provide an \"Are you sure\" dialog (or some other notification) before the application exits, place that code here. This message is typically sent from a Panel Close? event."
        # "Confirm Quit - Message that can confirm whether or not the user wants to exit the application."
        n859 = call-poly "Enqueue Message.vi"("Priority Message? (F)"=TRUE, "error in (no error)"=w1070, "Message"="Exit", "Message Queue"=w1066) -> ("error out"=w1067:errorcluster)  [unwired: 6 in, 1 out]
        n860 = Merge Errors(w1067) -> (w1068:errorcluster)
      }
      frame "Exit" {
        # "Stop the VI"
        # "Release the message queue reference"
        # "#CodeNeeded - Add any required cleanup code here. Note that if 'Exit' was called as a result of an error, an error dialog will be displayed. Add any custom error handling for an 'Exit' condition here as well."
        # "Exit - Exit the application."
        n861 = call "Fire User Event - Stop.vi"("User Event - Stop"=w1071) -> ("error out"=w1073:errorcluster)  [unwired: 10 in]
        n862 = Release Queue(queue=w1078, error in (no error)=w1072) -> (error out=w1075:errorcluster)  [unwired: 1 in, 2 out]
        n863 = Merge Errors(w1073, w1075) -> (w1074:errorcluster)
      }
      frame Default {
        # "'Default' case only runs if there is a message that isn't defined in any of the other cases.  Output a programming error."
        n864 = xnode ("Error Ring")("parameter 0"=w1079) -> ("error out"=w1080:errorcluster)
      }
    }
    n865 = Unbundle By Name(w1015) -> ("Environmental control.Acoustic Emission 3"=w1023:refnum<vi>)
    n866 = call "LAB-IQ Error Handler - Message Handling Loop.vi"("error in (no error)"=w1027, "Message Queue"=w1029) -> ("dup error in"=w1028:errorcluster)  [unwired: 8 in, 1 out]
    n867 = property on="Property Node" class="Bool (strict)"(reference=w1023) -> (reference out=w1021:refnum<vi>, error out=w1022:errorcluster, "Value"=w1020:bool)  [unwired: 1 in]
